vi "MTMount_getSample_OSS.vi"(8 "error in (no error)":errorcluster, 11 "OSS_Ctl":T1) -> (0 "error out":errorcluster, 2 "function return":i32, 3 "OSS_Ctl out":T1)   [LabVIEW 2018, in "SALLV_MTMount.lvlib"]
doc: "int MTMount_shm_getSample_OSSLV(MTMount_OSSLV *OSS_Ctl );"
uses:
  SALLV_MTMount.lvlib
  DataTypes/OSS.ctl
  SALLV_MTMount.so
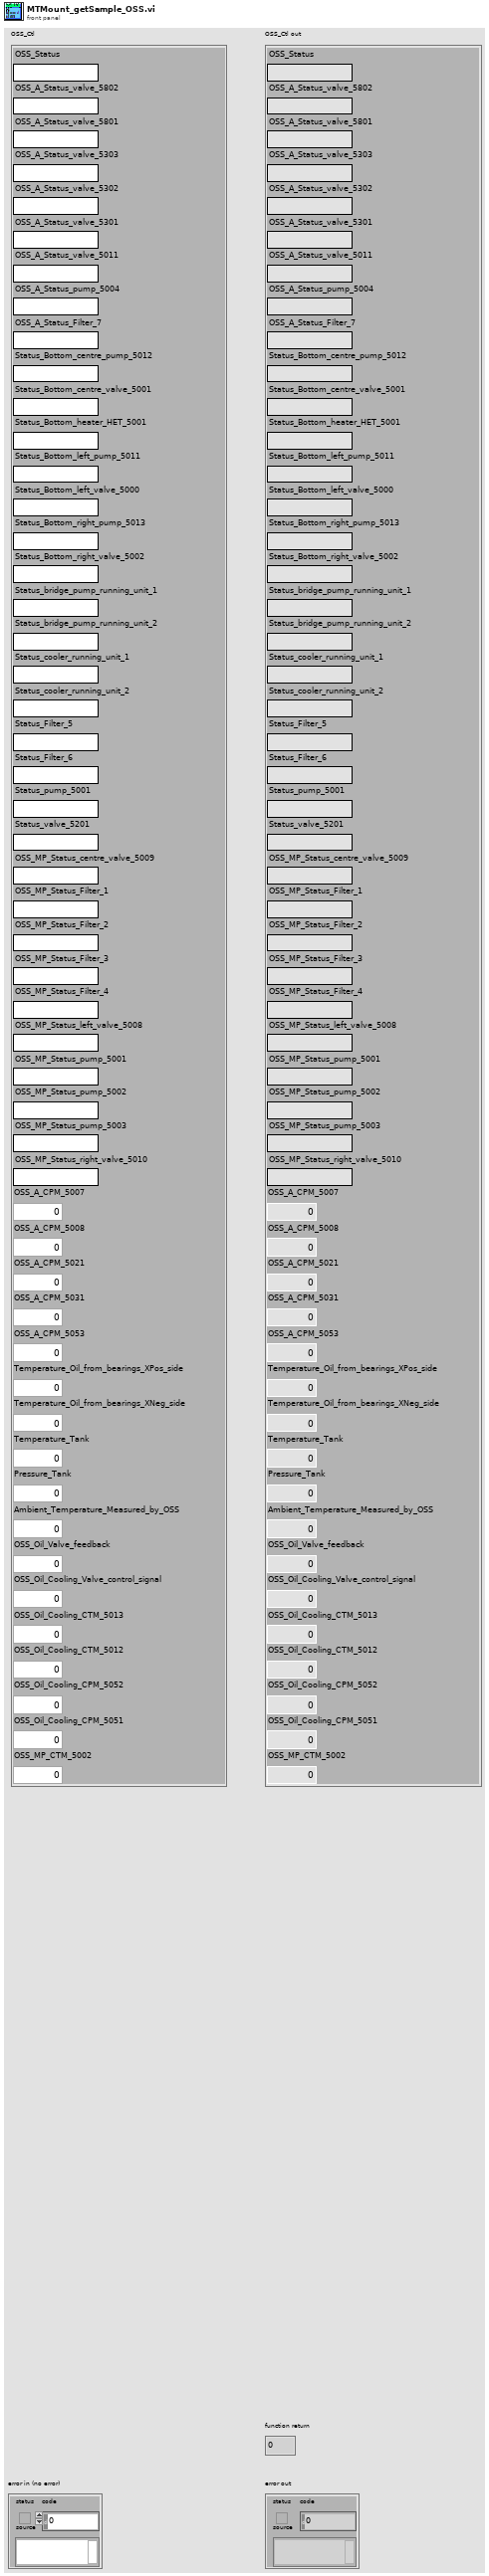
[diagram p1: front panel]
types:
  T1 = typedef "SALLV_MTMount.lvlib/OSS.ctl" = cluster{"OSS_Status":string, "OSS_A_Status_valve_5802":string, "OSS_A_Status_valve_5801":string, "OSS_A_Status_valve_5303":string, "OSS_A_Status_valve_5302":string, "OSS_A_Status_valve_5301":string, "OSS_A_Status_valve_5011":string, "OSS_A_Status_pump_5004":string, "OSS_A_Status_Filter_7":string, "Status_Bottom_centre_pump_5012":string, "Status_Bottom_centre_valve_5001":string, "Status_Bottom_heater_HET_5001":string, "Status_Bottom_left_pump_5011":string, "Status_Bottom_left_valve_5000":string, "Status_Bottom_right_pump_5013":string, "Status_Bottom_right_valve_5002":string, "Status_bridge_pump_running_unit_1":string, "Status_bridge_pump_running_unit_2":string, "Status_cooler_running_unit_1":string, "Status_cooler_running_unit_2":string, "Status_Filter_5":string, "Status_Filter_6":string, "Status_pump_5001":string, "Status_valve_5201":string, "OSS_MP_Status_centre_valve_5009":string, "OSS_MP_Status_Filter_1":string, "OSS_MP_Status_Filter_2":string, "OSS_MP_Status_Filter_3":string, "OSS_MP_Status_Filter_4":string, "OSS_MP_Status_left_valve_5008":string, "OSS_MP_Status_pump_5001":string, "OSS_MP_Status_pump_5002":string, "OSS_MP_Status_pump_5003":string, "OSS_MP_Status_right_valve_5010":string, "OSS_A_CPM_5007":dbl, "OSS_A_CPM_5008":dbl, "OSS_A_CPM_5021":dbl, "OSS_A_CPM_5031":dbl, "OSS_A_CPM_5053":dbl, "Temperature_Oil_from_bearings_XPos_side":dbl, "Temperature_Oil_from_bearings_XNeg_side":dbl, "Temperature_Tank":dbl, "Pressure_Tank":dbl, "Ambient_Temperature_Measured_by_OSS":dbl, "OSS_Oil_Valve_feedback":dbl, "OSS_Oil_Cooling_Valve_control_signal":dbl, "OSS_Oil_Cooling_CTM_5013":dbl, "OSS_Oil_Cooling_CTM_5012":dbl, "OSS_Oil_Cooling_CPM_5052":dbl, "OSS_Oil_Cooling_CPM_5051":dbl, "OSS_MP_CTM_5002":dbl}
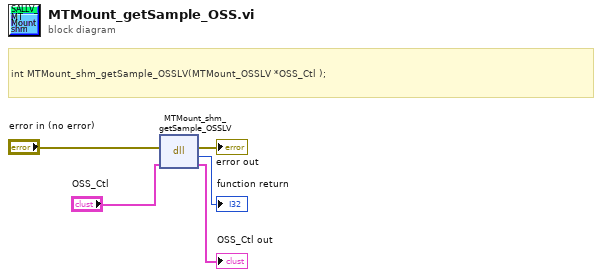
[diagram p0: block diagram]
diagram:
  # "int MTMount_shm_getSample_OSSLV(MTMount_OSSLV *OSS_Ctl );"
  n1 = dll-call lib="home/ttsai/Document/salApiMTMount/SALLV_MTMount/SALLV_MTMount.*" fn="MTMount_shm_getSample_OSSLV"(error in="error in (no error)", "OSS_Ctl"="OSS_Ctl") -> (error out=→"error out":errorcluster, →"function return":i32, "OSS_Ctl"=→"OSS_Ctl out":T1)  [unwired: 2 in, 1 out]
